vi "Node Contants.vi"(8 "error in (no error)":errorcluster) -> (0 "error out":errorcluster, 2 "Constants":T1)   [LabVIEW 2019, in "Node.lvclass"]
uses:
  Node.lvclass
  Shared/Node Type--enum.ctl
  Node.lvclass/Node.ctl
  Shared/Shared.lvlib
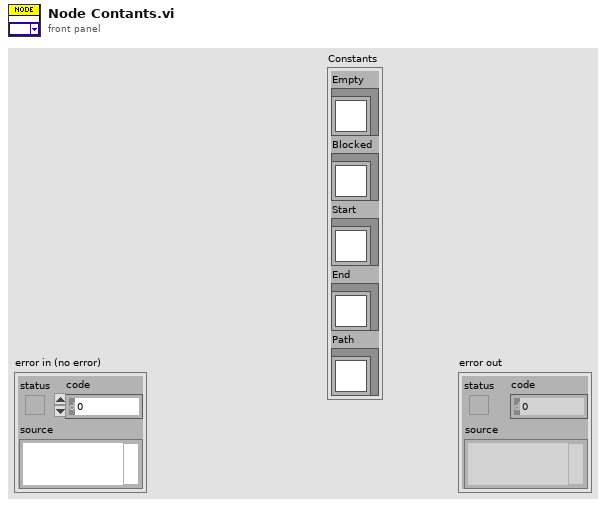
[diagram p1: front panel]
types:
  T1 = cluster{"Empty":refnum<class "Node.lvclass">, "Blocked":refnum<class "Node.lvclass">, "Start":refnum<class "Node.lvclass">, "End":refnum<class "Node.lvclass">, "Path":refnum<class "Node.lvclass">}
  T2 = typedef "Shared.lvlib/Node Type--enum.ctl" = enum16{"Empty", "Blocked", "Start", "End", "Path"}
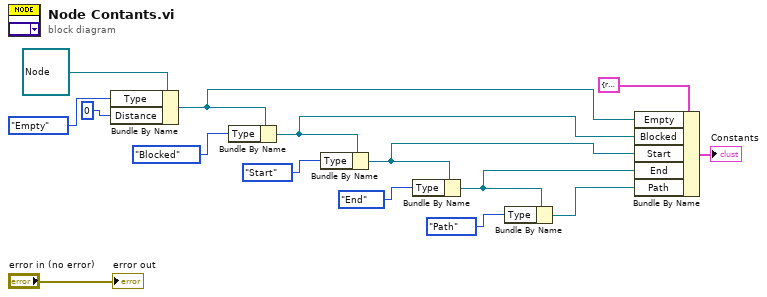
[diagram p0: block diagram]
diagram:
  n1 = Bundle By Name(cluster=refnum<class "Node.lvclass"> refnum ("Picture Ring.lvclass"), "Type"=Node_Type--enum."Empty", "Distance"=0) -> (w7:refnum<class "Node.lvclass">)
  n2 = Bundle By Name(cluster=w7, "Type"=Node_Type--enum."Blocked") -> (w6:refnum<class "Node.lvclass">)
  n3 = Bundle By Name(cluster=w6, "Type"=Node_Type--enum."Start") -> (w5:refnum<class "Node.lvclass">)
  n4 = Bundle By Name(cluster=w5, "Type"=Node_Type--enum."End") -> (w4:refnum<class "Node.lvclass">)
  n5 = Bundle By Name(cluster=w4, "Type"=Node_Type--enum."Path") -> (w3:refnum<class "Node.lvclass">)
  n6 = Bundle By Name(cluster=T1 {"Empty"=refnum, "Blocked"=refnum, "Start"=refnum, "End"=refnum, "Path"=refnum} ("Constants"), "Empty"=w7, "Blocked"=w6, "Start"=w5, "End"=w4, "Path"=w3) -> (→"Constants":T1)
  "error out" <- "error in (no error)"
